vi "Scan Setup.vi"(8 "error in (no error)":errorcluster, 11 "Microwave Freq Scan in":refnum<class "Microwave Freq Scan.lvclass">) -> (0 "error out":errorcluster, 3 "Microwave Freq Scan out":refnum<class "Microwave Freq Scan.lvclass">)   [LabVIEW 2009, in "Microwave Freq Scan.lvclass"]
doc: "Configure the instrument based on the class member data. This step comes after the user has closed the \"Scan Setup\" window and before the actual scan -- so instruments are configured with the user's specified settings."
uses:
  Microwave Freq Scan.lvclass
  Scanner/Scanner.lvclass
  Instruments/Utility Classes/Scannable/Scannable.lvclass
  Microwave Freq Scan.lvclass/Microwave Freq Scan.ctl
  Instruments/Microwave/Agilent PSG MXG Series/Agilent PSG MXG Series.lvlib
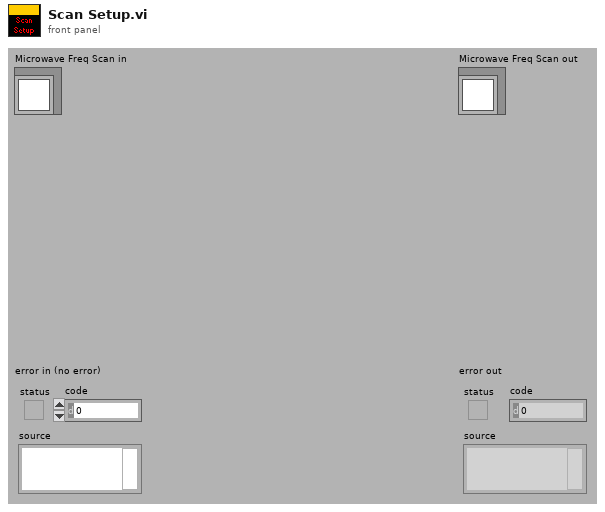
[diagram p1: front panel]
types:
  T1 = enum16{"CW", "Fixed", "Stepped Sweep", "List Sweep"}
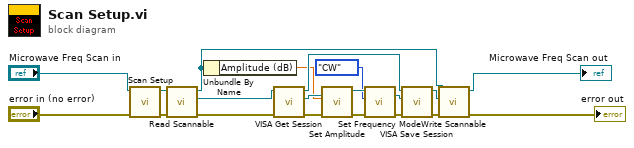
[diagram p0: block diagram]
diagram:
  n1 = call-parent "Scan Setup.vi"("error in (no error)"="error in (no error)", "Scanner in"="Microwave Freq Scan in") -> ("error out"=w5:errorcluster, "Scanner out"=w6:refnum<class "Microwave Freq Scan.lvclass">)  [unwired: 8 out]
  n2 = call-dynamic "Read Scannable.vi"("error in (no error)"=w5, "Scanner.lvclass in"=w6) -> ("error out"=w18:errorcluster, "Scannable.lvclass"=w17:refnum<class "Scannable.lvclass">, "Scanner.lvclass out"=w4:refnum<class "Microwave Freq Scan.lvclass">)  [unwired: 7 out]
  n3 = Unbundle By Name(w4) -> ("Amplitude (dB)"=w3:dbl)
  n4 = call-dynamic "VISA Get Session.vi"("error in (no error)"=w18, "Instrument.lvclass in"=w17) -> ("error out"=w9:errorcluster, "VISA Resource Name"=w13:refnum<visa-resource-name>, "Instrument.lvclass out"=w12:refnum<class "Scannable.lvclass">)  [unwired: 7 out]
  n5 = call "Set Amplitude.vi"("error in (no error)"=w9, "Amplitude (dBm)"=w3, "VISA resource name"=w13) -> ("error out"=w8:errorcluster, "VISA resource name out"=w11:refnum<visa-resource-name>)  [unwired: 7 out]
  n6 = call "Set Frequency Mode.vi"("error in (no error)"=w8, "Frequency Mode"=T1."CW", "VISA resource name"=w11) -> ("error out"=w7:errorcluster, "VISA resource name out"=w10:refnum<visa-resource-name>)  [unwired: 7 out]
  n7 = call-dynamic "VISA Save Session.vi"("error in (no error)"=w7, "VISA Resource Name"=w10, "Instrument.lvclass in"=w12) -> ("error out"=w16:errorcluster, "Instrument.lvclass out"=w1:refnum<class "Scannable.lvclass">)  [unwired: 7 out]
  n8 = call-dynamic "Write Scannable.vi"("error in (no error)"=w16, "Scannable.lvclass"=w1, "Scanner.lvclass in"=w4) -> ("error out"=→"error out":errorcluster, "Scanner.lvclass out"=→"Microwave Freq Scan out":refnum<class "Microwave Freq Scan.lvclass">)  [unwired: 7 out]
